vi "RT 16 bit ADC DAC_KA1.vi"() -> ()   [LabVIEW 2018]
uses:
  <vilib>/rvi/interface/nirviCloseFPGA/nirviCloseFPGA.xnode
  <vilib>/FPGAPlugInAG/Dynamic/niLvFpga_Close_Dynamic.vi
  <vilib>/rvi/interface/nirviOpenFPGA/nirviOpenFPGA.xnode
  FPGA Bitfiles/ASPE2019StudentC_FPGATarget_FPGASPI_ZCDGpJzZuc4.lvbitx
  16Bit_ADC_DAC/FPGA_SPI.vi
  <vilib>/FPGAPlugInAG/myRIO-1900/niLvFpga_Open_myRIO-1900.vi
  <vilib>/rvi/interface/common/dynamic/niFpgaDynamicAddResources.vi
panel:
  in  "stop":bool
  in  "samples per cycle":u32=1000
  in  "Amplitude":dbl=1.0 format="%0.3p"
  in  "time delay":u32=1
  out "avg. loop rate (kHz)":dbl format="%#_2g"
  in  "CH1":bool[](array[boolean])=[FALSE, FALSE, TRUE, FALSE, FALSE, TRUE, FALSE, FALSE, FALSE, FALSE, FALSE, FALSE, FALSE, FALSE, FALSE, FALSE]
  in  "CH3":bool[](array[boolean])=[FALSE, FALSE, FALSE, TRUE, FALSE, TRUE, FALSE, FALSE, FALSE, FALSE, FALSE, FALSE, FALSE, FALSE, FALSE, FALSE]
  in  "CH2":bool[](array[boolean])=[FALSE, FALSE, FALSE, FALSE, FALSE, TRUE, FALSE, FALSE, FALSE, FALSE, FALSE, FALSE, FALSE, FALSE, FALSE, FALSE]
  out "Cap probe":dbl(graph)=0.00030517112470818
  out "EMF (Velocity mode)":dbl(graph)
  out "sense (Force mode)":dbl(graph)
  in  "Color Box":u32(colorbox)
  in  "?":u32(colorbox)
  # "Force mode"
  # "Velocity mode"
  # "DAC"
  # "ADC"
  # "when you write to channel 2 of ADC, \nyou read previous channel (ch 1 to which cap probe is connected to)  \nRef:Table 1,2: ADC LTC1859"
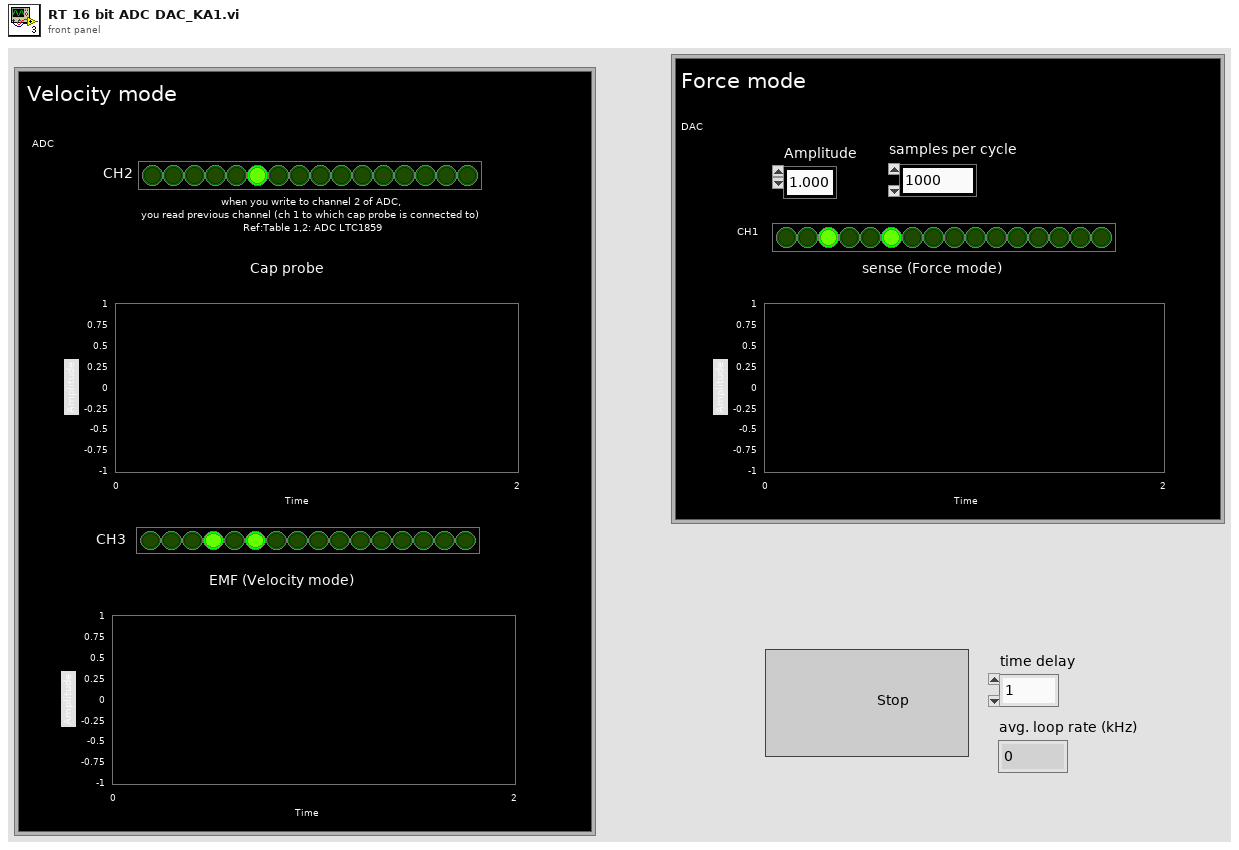
[diagram p1: front panel]
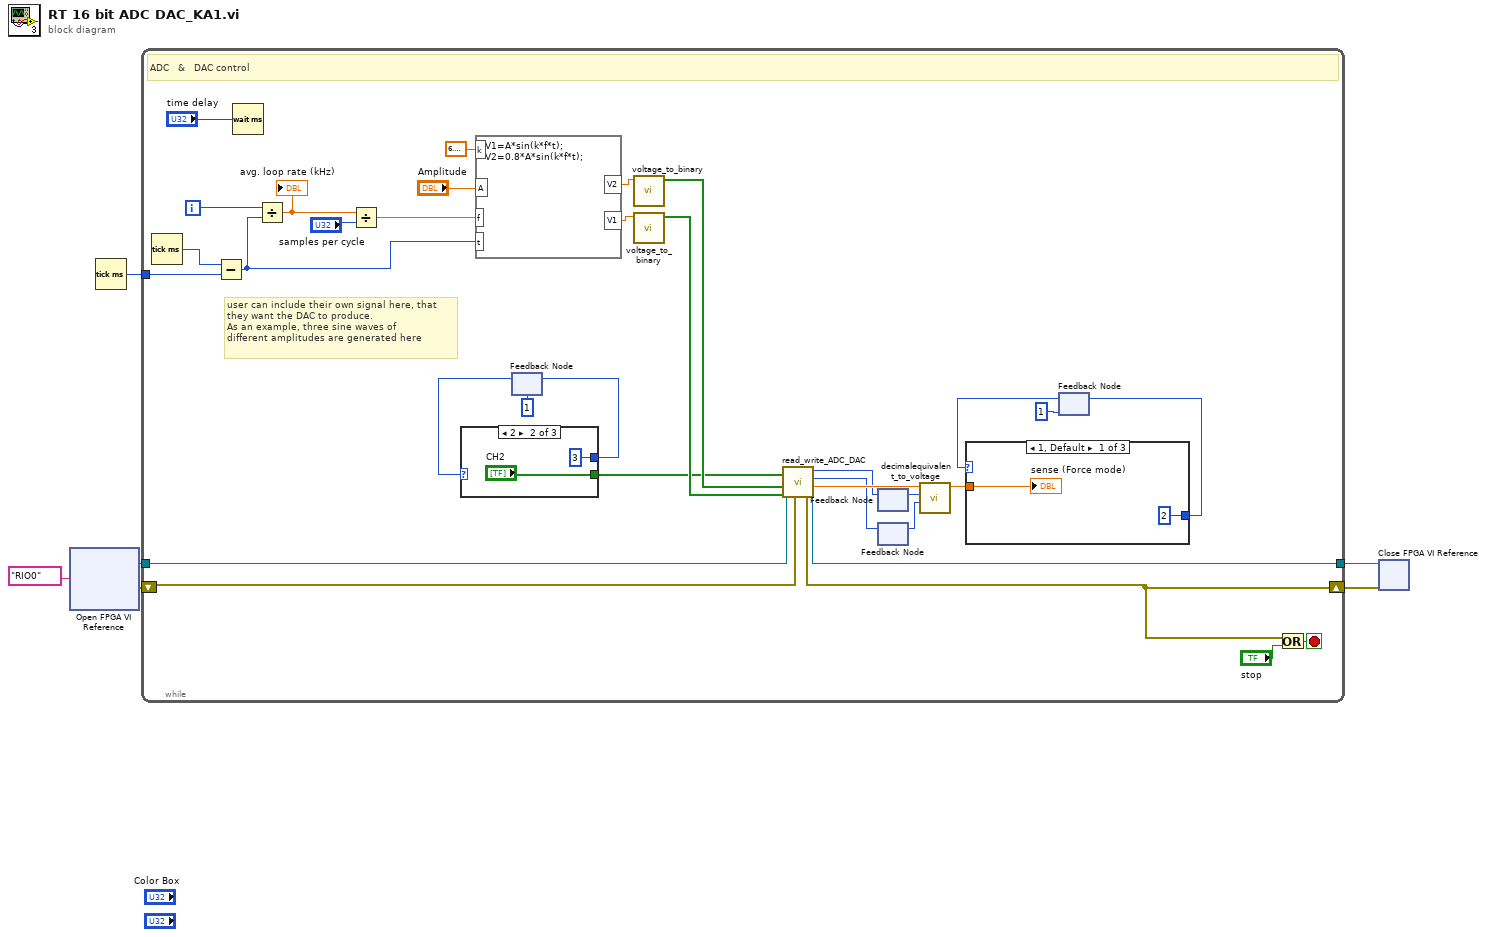
[diagram p0: block diagram]
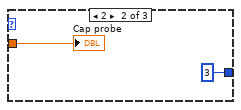
[diagram p2: hidden frame]
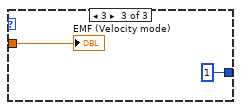
[diagram p3: hidden frame]
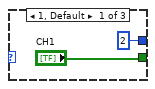
[diagram p4: hidden frame]
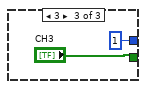
[diagram p5: hidden frame]
diagram:
  n1 = xnode "Open FPGA VI Reference"("resource name"=tag "RIO0") -> ("FPGA VI Reference Out"=w5:refnum<k20>, "error out"=w4:errorcluster)  [unwired: 1 in]
  n2 = Tick Count (ms)() -> (millisecond timer value=w2:u32)
  n3 = while {
    shift-right: [w20] -> w6
    shift-left: w4 -> [w25]
    tunnel: w2 -> [w37]
    tunnel: w5 -> [w26]
    tunnel: [w21] -> w1
    i -> [w19]
    stop <- w38 stop-if-true
    # "user can include their own signal here, that \nthey want the DAC to produce.\nAs an example, three sine waves of \ndifferent amplitudes are generated here"
    # "ADC   &   DAC control"
    n4 = Tick Count (ms)() -> (millisecond timer value=w35:u32)
    n5 = Subtract(x=w35, y=w37) -> (x-y=w29:u32)
    n6 = Wait (ms)(milliseconds to wait="time delay") -> ()  [unwired: 1 out]
    n7 = Divide(x=w19, y=w29) -> (x/y=w34:dbl)
    "avg. loop rate (kHz)" <- w34
    n8 = Divide(x=w34, y="samples per cycle") -> (x/y=w31:dbl)
    n9 = formula code="V1=A*sin(k*f*t);\nV2=0.8*A*sin(k*f*t);"("t"=w29, "f"=w31, "A"="Amplitude", "k"=6.283185307179586 ("input variable")) -> ("V1"=w28:dbl, "V2"=w27:dbl)
    n10 = feedback #1(1) -> (w17:i32)
    n11 = case shown="2" w17 {
      tunnel: ["CH1" "CH2" "CH3"] -> w15
      tunnel: [2 3 1] -> w18
      frame 1, Default {
      }
      frame 2 {
      }
      frame 3 {
      }
    }
    n12 = feedback-in #1(w18) -> ()
    n13 = call "voltage_to_binary.vi"("voltage"=w27) -> ("binary"=w24:bool[])  [unwired: 10 in]
    n14 = call "voltage_to_binary.vi"("voltage"=w28) -> ("binary"=w23:bool[])  [unwired: 10 in]
    n15 = call "read_write_ADC_DAC.vi"("CH"=w15, "DAC2"=w23, "DAC1"=w24, "error in"=w25, "FPGA VI Reference In"=w26) -> ("FPGA VI Reference Out"=w21:refnum<k20>, "i"=w22:dbl, "GAIN"=w11:i16, "UNI"=w13:i16, "error out"=w20:errorcluster)  [unwired: 2 in]
    n16 = feedback-in #2(w13) -> ()
    n17 = feedback #2() -> (w12:i16)  [unwired: 1 in]
    n18 = feedback #3() -> (w10:i16)  [unwired: 1 in]
    n19 = feedback-in #3(w11) -> ()
    n20 = call "decimalequivalent_to_voltage.vi"("GAIN"=w10, "UNI"=w12, "i"=w22) -> ("V"=w14:dbl)  [unwired: 8 in]
    n21 = feedback #4(1) -> (w8:i32)
    n22 = case shown="1, Default" w8 {
      tunnel: [2 3 1] -> w9
      tunnel: w14 -> [w40 w42 w44]
      frame 1, Default {
        "sense (Force mode)" <- w40
      }
      frame 2 {
        "Cap probe" <- w42
      }
      frame 3 {
        "EMF (Velocity mode)" <- w44
      }
    }
    n23 = feedback-in #4(w9) -> ()
    n24 = Or(x=w20, y="stop") -> (x .or. y?=w38:bool)
  }
  n25 = xnode "Close FPGA VI Reference"("FPGA VI Reference In"=w1, "error in"=w6) -> ()  [unwired: 1 out]
